vi "tp4-3.vi"() -> ()   [LabVIEW 2013]
panel:
  out "XY Graph":cluster{dbl[], dbl[]}[](graph)
  in  "Frecuencia":dbl=150.0
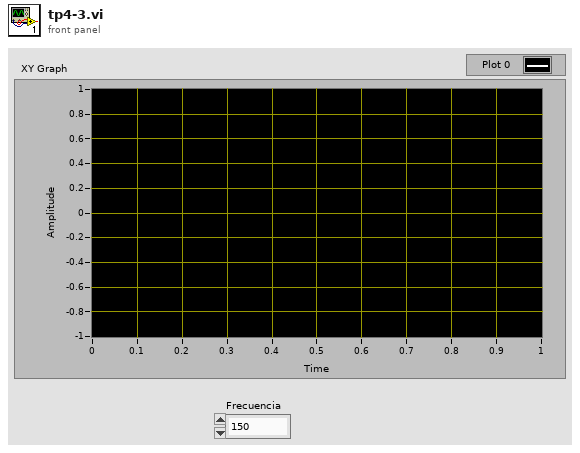
[diagram p1: front panel]
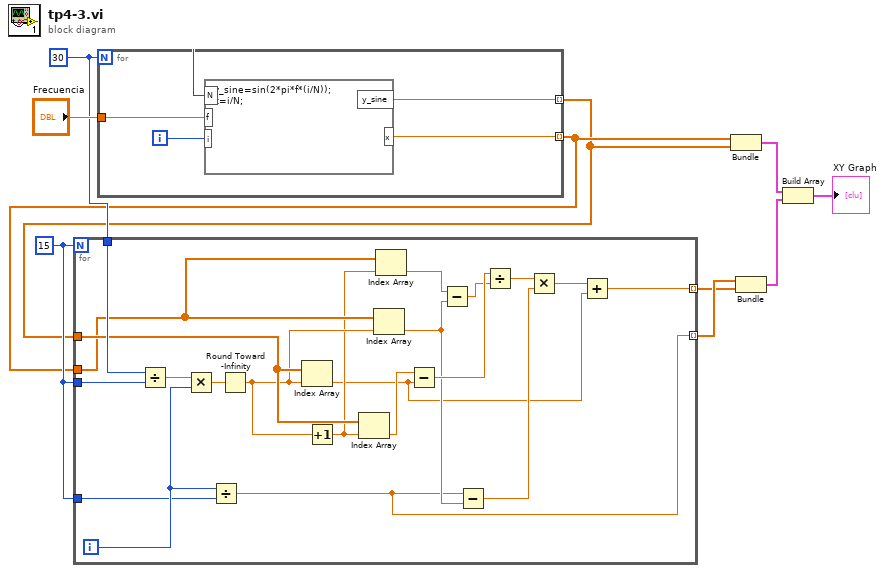
[diagram p0: block diagram]
diagram:
  w8 = 15
  w9 = 30
  n1 = for {
    N: w9 -> [w15]
    tunnel: "Frecuencia" -> [w14]
    tunnel: [w13] -> w6 mode=indexing
    tunnel: [w12] -> w7 mode=indexing
    i -> [w11]
    n2 = formula code="y_sine=sin(2*pi*f*(i/N));\nx=i/N;"("i"=w11, "N"=w15, "f"=w14) -> ("y_sine"=w13:dbl, "x"=w12:dbl)
  }
  n3 = for {
    N: w8 -> [_]
    tunnel: w6 -> [w32]
    tunnel: w7 -> [w30]
    tunnel: w8 -> [w36]
    tunnel: w9 -> [w35]
    tunnel: w8 -> [w23]
    tunnel: [w18] -> w4 mode=indexing
    tunnel: [w16] -> w5 mode=indexing
    i -> [w24]
    n4 = Divide(x=w35, y=w36) -> (x/y=w34:dbl)
    n5 = Multiply(x=w34, y=w24) -> (x*y=w33:dbl)
    n6 = Divide(x=w24, y=w23) -> (x/y=w16:dbl)
    n7 = Round Toward -Infinity(1:w33) -> (0:w31:dbl)
    n8 = Index Array(array=w32, index=w31) -> (element=w17:dbl)
    n9 = Increment(x=w31) -> (x+1=w29:dbl)
    n10 = Index Array(array=w32, index=w29) -> (element=w19:dbl)
    n11 = Index Array(array=w30, index=w31) -> (element=w22:dbl)
    n12 = Index Array(array=w30, index=w29) -> (element=w28:dbl)
    n13 = Subtract(x=w19, y=w17) -> (x-y=w27:dbl)
    n14 = Subtract(x=w28, y=w22) -> (x-y=w26:dbl)
    n15 = Subtract(x=w16, y=w22) -> (x-y=w21:dbl)
    n16 = Divide(x=w27, y=w26) -> (x/y=w25:dbl)
    n17 = Multiply(x=w25, y=w21) -> (x*y=w20:dbl)
    n18 = Add(x=w20, y=w17) -> (x+y=w18:dbl)
  }
  n19 = Bundle(w7, w6) -> (w3:cluster{dbl[], dbl[]})  [unwired: 1 in]
  n20 = Bundle(w5, w4) -> (w2:cluster{dbl[], dbl[]})  [unwired: 1 in]
  n21 = Build Array(w3, w2) -> (→"XY Graph":cluster{dbl[], dbl[]}[])
